vi "Update Description map.vi"(7 "Item":string, 10 "Description":string, 11 "Test Tree In":refnum<class "Test Tree.lvclass">) -> (3 "Test Tree Out":refnum<class "Test Tree.lvclass">)   [LabVIEW 2020, in "Test Tree.lvclass"]
uses:
  Test Tree.lvclass
  Test Tree.lvclass/Test Tree.ctl
  <vilib>/Utility/miscctls.llb/LVMapReplaceAction.ctl
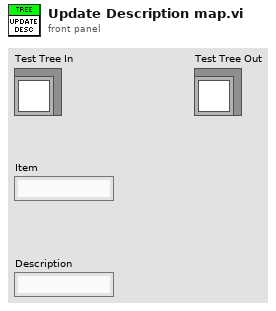
[diagram p1: front panel]
types:
  T1 = typedef "LVMapReplaceAction.ctl" = enum32{"Modify Entry only if found", "Add or Modify Entry", "Delete Entry"}
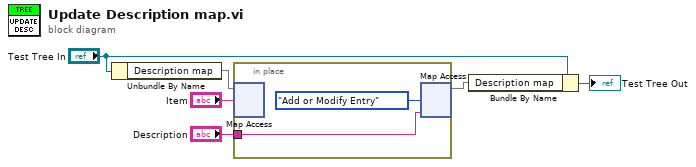
[diagram p0: block diagram]
diagram:
  n1 = Unbundle By Name("Test Tree In") -> ("Description map"=w5:map{string, string})
  n2 = in-place {
    in-place-border: "Description" -> [w8]
    n3 = in-place-map #1(w5, "Item") -> ()  [unwired: 1 in, 2 out]
    n4 = in-place-map #1(w8, LVMapReplaceAction."Add or Modify Entry" ("action")) -> (w1:map{string, string})  [unwired: 2 out]
  }
  n5 = Bundle By Name(cluster="Test Tree In", "Description map"=w1) -> (→"Test Tree Out":refnum<class "Test Tree.lvclass">)
